vi "04-Vending2.vi"() -> ()   [LabVIEW 2017]
uses:
  Support/03-Typedef.ctl
panel:
  in  "100 Yen":bool
  in  "Change":bool
  out "Current Value":i32
  in  "Vend":bool
  in  "stop":bool
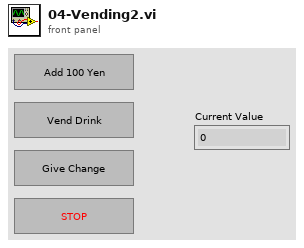
[diagram p1: front panel]
types:
  T1 = typedef "03-Typedef.ctl" = enum16{"Init", "Vend", "Change", "Add Money", "Idle", "Exit"}
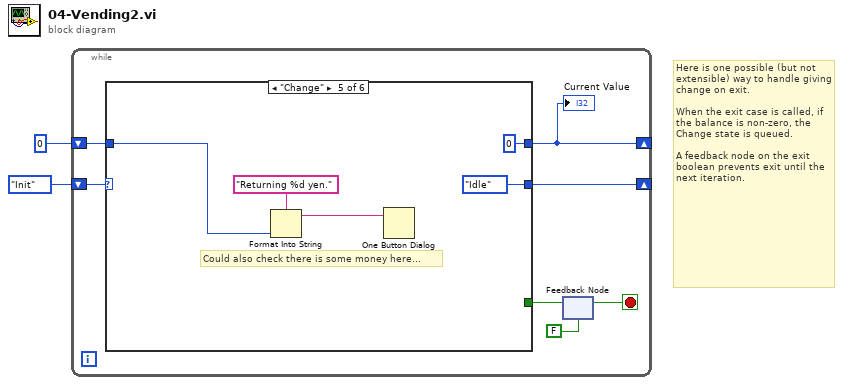
[diagram p0: block diagram]
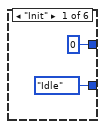
[diagram p2: hidden frame]
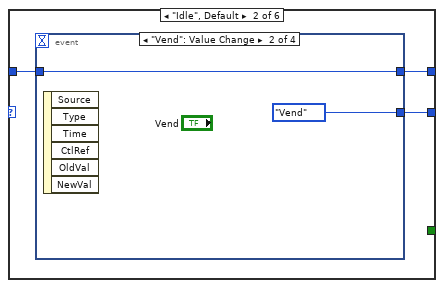
[diagram p3: hidden frame]
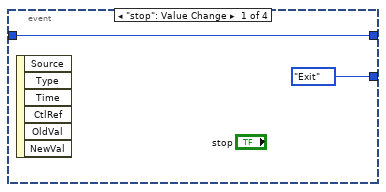
[diagram p4: hidden frame]
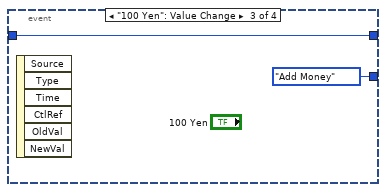
[diagram p5: hidden frame]
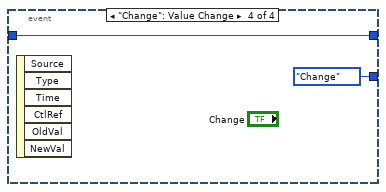
[diagram p6: hidden frame]
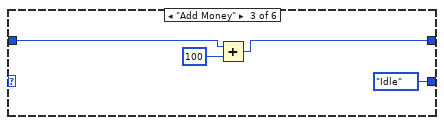
[diagram p7: hidden frame]
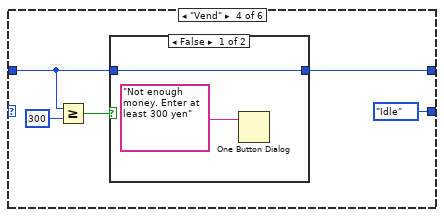
[diagram p8: hidden frame]
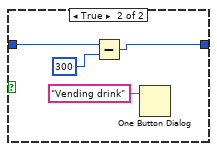
[diagram p9: hidden frame]
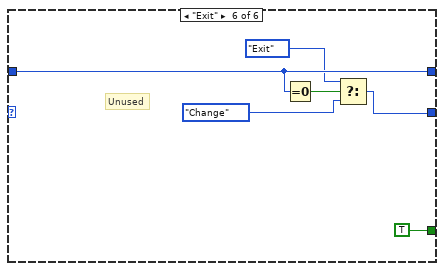
[diagram p10: hidden frame]
diagram:
  # "Here is one possible (but not extensible) way to handle giving change on exit.\n\nWhen the exit case is called, if the balance is non-zero, the Change state is queued. \n\nA feedback node on the exit boolean prevents exit until the next iteration."
  n1 = while {
    shift-right: [w7] -> _
    shift-left: 03-Typedef."Init" ("Enum") -> [w9]
    shift-right: [w5] -> _
    shift-left: 0 -> [w6]
    stop <- w4 stop-if-true
    n2 = case shown="\"Change\"" w9 {
      tunnel: [_ _ _ _ _ TRUE] -> w8
      tunnel: [03-Typedef."Idle" ("Enum") w14 03-Typedef."Idle" ("Enum") 03-Typedef."Idle" ("Enum") 03-Typedef."Idle" ("Enum") w43] -> w7
      tunnel: w6 -> [_ w13 w26 w28 w40 w47]
      tunnel: [0 w12 w25 w27 0 w47] -> w5
      frame "Init" {
      }
      frame "Idle", Default {
        n3 = event shown="[1] \"Vend\": Value Change" {
          selector: _ -> [_ _ _ _]
          dyn-events: _ -> [_ _ _ _]
          timeout: _ -> [_ _ _ _]
          tunnel: [03-Typedef."Exit" ("t") 03-Typedef."Vend" ("Enum") 03-Typedef."Add Money" ("Enum") 03-Typedef."Change" ("Enum")] -> w14
          tunnel: w13 -> [w15 w17 w19 w22]
          tunnel: [w15 w17 w19 w22] -> w12
          event "stop": Value Change {
            n4 = event-data() -> ()  [unwired: 1 in, 6 out]
          }
          event "Vend": Value Change {
            n5 = event-data() -> ()  [unwired: 1 in, 6 out]
          }
          event "100 Yen": Value Change {
            n6 = event-data() -> ()  [unwired: 1 in, 6 out]
          }
          event "Change": Value Change {
            n7 = event-data() -> ()  [unwired: 1 in, 6 out]
          }
        }
      }
      frame "Add Money" {
        n8 = Add(x=w26, y=100) -> (x+y=w25:i32)
      }
      frame "Vend" {
        n9 = Greater Or Equal?(x=w28, y=300) -> (x >= y?=w29:bool)
        n10 = case shown="False" w29 {
          tunnel: w28 -> [w32 w36]
          tunnel: [w32 w34] -> w27
          frame False {
            n11 = One Button Dialog(message="Not enough money. Enter at least 300 yen") -> ()  [unwired: 1 in, 1 out]
          }
          frame True {
            n12 = Subtract(x=w36, y=300) -> (x-y=w34:i32)
            n13 = One Button Dialog(message="Vending drink") -> ()  [unwired: 1 in, 1 out]
          }
        }
      }
      frame "Change" {
        # "Could also check there is some money here..."
        n14 = Format Into String(format string="Returning %d yen.", w40) -> (resulting string=w41:string)  [unwired: 2 in, 1 out]
        n15 = One Button Dialog(message=w41) -> ()  [unwired: 1 in, 1 out]
      }
      frame "Exit" {
        # "Unused"
        n16 = Equal To 0?(x=w47) -> (x = 0?=w46:bool)
        n17 = Select(t=03-Typedef."Exit" ("Enum"), s=w46, f=03-Typedef."Change" ("Enum")) -> (s? t:f=w43:T1)
      }
    }
    "Current Value" <- w5
    n18 = feedback-in #1(w8) -> ()
    n19 = feedback #1(FALSE) -> (w4:bool)
  }
